vi "Main.vi"() -> ()   [LabVIEW 2015]
uses:
  <vilib>/myRIO/Instrument Drivers/Onboard IO/DIO/typedefs/DIO Reference.ctl
  <vilib>/myRIO/Common/Instrument Driver Framework/Utilities/typedefs/myRIO Generic Hardware Reference.ctl
  <vilib>/myRIO/Common/Instrument Driver Framework/Utilities/typedefs/Hardware Version Enum.ctl
  <vilib>/myRIO/Common/Instrument Driver Framework/Utilities/typedefs/myRIO v1.0 Reference.ctl
  <vilib>/myRIO/Common/Instrument Driver Framework/Utilities/typedefs/Generic FPGA Reference.ctl
  <vilib>/myRIO/Common/Instrument Driver Framework/myRIO v1.0/DIO/typedefs/DIO Channels List.ctl
  <vilib>/myRIO/Common/Instrument Driver Framework/myRIO v1.0/DIO/typedefs/DIO Channels Enum.ctl
  <vilib>/userdefined/High Color/nirio_resource_hc.ctl
  <vilib>/myRIO/Common/Instrument Driver Framework/Utilities/vis/Is FPGA Ref Available.vi
  <vilib>/myRIO/Common/Instrument Driver Framework/myRIO v1.0/DIO/vis/myRIO v1.1 Open DIO.vi
  <vilib>/myRIO/Instrument Drivers/Onboard IO/DIO/vis/Write.vi
  <vilib>/myRIO/Common/Instrument Driver Framework/Utilities/vis/Validate Channels.vi
  <vilib>/myRIO/Common/Instrument Driver Framework/myRIO v1.0/DIO/vis/myRIO v1.0 Reserve DIO.vi
  <vilib>/myRIO/Common/Instrument Driver Framework/myRIO v1.0/Resource Manager/vis/myRIO v1.0 Reserve Channel List.vi
  <vilib>/myRIO/Common/Instrument Driver Framework/myRIO v1.0/DIO/vis/myRIO v1.0 Build MUX Configuration DIO.vi
  <vilib>/myRIO/Common/Instrument Driver Framework/myRIO v1.0/Resource Manager/vis/myRIO v1.0 Reserve Channel.vi
  <vilib>/myRIO/Common/Instrument Driver Framework/myRIO v1.0/Resource Manager/vis/myRIO v1.0 Unreserve Channel.vi
  <vilib>/myRIO/Common/Instrument Driver Framework/myRIO v1.0/Resource Manager/vis/myRIO v1.0 Create Configuration List.vi
  <vilib>/myRIO/Common/Instrument Driver Framework/myRIO v1.0/Resource Manager/vis/myRIO v1.0 Build Mutex Name.vi
  <vilib>/Utility/VariantDataType/GetNumericInfo.vi
  <vilib>/Utility/error.llb/Error Cluster From Error Code.vi
  <vilib>/myRIO/Common/Instrument Driver Framework/myRIO v1.0/myRIO v1.1 Open.vi
  <vilib>/myRIO/Common/Instrument Driver Framework/Utilities/vis/IO Manager.vi
  <vilib>/myRIO/Common/Instrument Driver Framework/Utilities/vis/Configuration Manager.vi
  <vilib>/myRIO/Common/Instrument Driver Framework/myRIO v1.0/Resource Manager/vis/myRIO v1.0 Configure IO.vi
  <vilib>/myRIO/Common/Instrument Driver Framework/myRIO v1.0/myRIO v1.0 Close.vi
  <vilib>/myRIO/Common/Instrument Driver Framework/myRIO v1.0/DIO/vis/myRIO v1.0 Write DIO.vi
  <vilib>/myRIO/Express VI/Onboard Devices/LED/LED Express VI.xnode
  <vilib>/myRIO/Instrument Drivers/Onboard IO/DIO/vis/myRIO DIO Open.xnode
  <vilib>/myRIO/Express VI/Onboard IO/DO/DO Express VI.xnode
  <vilib>/myRIO/Instrument Drivers/Onboard IO/DIO/DIO.lvlib
panel:
  out "Image Out":T1(plugin-control)
  out "LMot":dbl(slide) scale=-1.0..1.0
  out "RMot":dbl(slide) scale=-1.0..1.0
  out "Translation Response":dbl
  out "Spin Response":dbl
  out "Y Axis Error":i32=100
  out "X Axis Error":i32=100
  out "Object Aquired":bool
  in  "stop":bool
  # "Robot Laser Tracker Main"
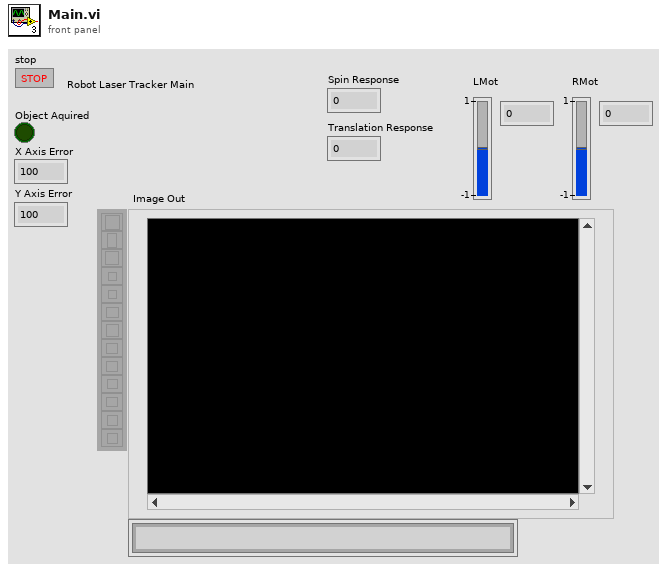
[diagram p1: front panel]
types:
  T1 = typedef "IMAQ Image.ctl" = refnum<image>
  T2 = typedef "DIO.lvlib/DIO Reference.ctl" = cluster{"myRIO Reference":T3, "DIO Channels List":T7}
  T3 = typedef "myRIO Generic Hardware Reference.ctl" = cluster{"myRIO Model":T4, "myRIO Hardware Reference":T5}
  T4 = typedef "Hardware Version Enum.ctl" = enum16{"Unknown", "myRIO-1900", "myRIO-1950", "roboRIO"}
  T5 = typedef "myRIO v1.0 Reference.ctl" = cluster{"Generic FPGA Reference":T6, "Allow multiple opens":bool}
  T6 = typedef "Generic FPGA Reference.ctl" = refnum<k20>
  T7 = typedef "DIO Channels List.ctl" = T8[]
  T8 = typedef "DIO Channels Enum.ctl" = enum16{"Not Connected", "C/DIO0", "C/DIO1", "C/DIO2", "C/DIO3", "C/DIO4", "C/DIO5", "C/DIO6", "C/DIO7", "A/DIO0", "A/DIO1", "A/DIO2", "A/DIO3", "A/DIO4", "A/DIO5", "A/DIO6", "A/DIO7", "A/DIO8", "A/DIO9", "A/DIO10", "A/DIO11", "A/DIO12", "A/DIO13", "A/DIO14", "A/DIO15", "B/DIO0", "B/DIO1", "B/DIO2", "B/DIO3", "B/DIO4", "B/DIO5", "B/DIO6", "B/DIO7", "B/DIO8", "B/DIO9", "B/DIO10", "B/DIO11", "B/DIO12", "B/DIO13", "B/DIO14", "B/DIO15", "LED0", "LED1", "LED2", "LED3", "Button0", "DIO/DIO0", "DIO/DIO1", "DIO/DIO2", "DIO/DIO3", "DIO/DIO4", "DIO/DIO5", "DIO/DIO6", "DIO/DIO7", "DIO/DIO8", "DIO/DIO9", "SPI/CS0", "SPI/CS1", "SPI/CS2", "SPI/CS3", "LED RADIO (Green)", "LED RADIO (Red)", "LED COMM (Green)", "LED COMM (Red)", "LED MODE (Green)", "LED MODE (Red)"}
  T9 = typedef "nirio_resource_hc.ctl" = tag
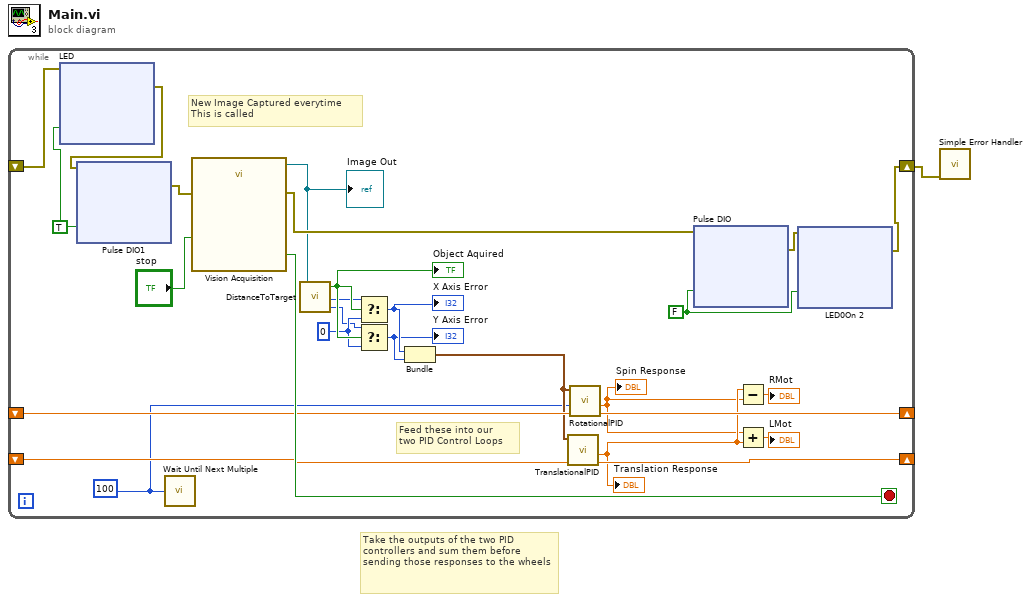
[diagram p0: block diagram]
diagram:
  # "Take the outputs of the two PID controllers and sum them before sending those responses to the wheels"
  n1 = while {
    shift-right: [w11] -> w1
    shift-left: _ -> [w14]
    shift-right: [w22] -> _
    shift-left: _ -> [w23]
    shift-right: [w21] -> _
    shift-left: _ -> [w20]
    stop <- w27 stop-if-true
    w5 = 0 ("f")
    w2 = u32 100 ("Tick Count(mSec)")
    w9 = FALSE ("A/DIO1 (Pin 13)")
    w12 = TRUE ("A/DIO1 (Pin 13)")
    # "New Image Captured everytime \nThis is called"
    # "Feed these into our \ntwo PID Control Loops"
    n2 = xnode "LED"("LED0"=w12, "error in (no error)"=w14) -> ("error out"=w13:errorcluster)
    n3 = xnode "Pulse DIO1"("A/DIO1 (Pin 13)"=w12, "error in (no error)"=w13) -> ("error out"=w28:errorcluster)
    n4 = call "Wait Until Next Multiple"("Count(mSec)"=w2) -> ()  [unwired: 1 out]
    n5 = call "Vision Acquisition"("Stop (F)"="stop", "error in"=w28) -> ("Image Out"=w24:T1, "Stopped"=w27:bool, "error out"=w25:errorcluster)  [unwired: 23 in]
    "Image Out" <- w24
    n6 = call "DistanceToTarget.vi"("Image Input"=w24) -> ("Y Axis Error"=w4:i32, "X Axis Error"=w6:i32, "Object Aquired"=w7:bool)  [unwired: 2 in]
    "Object Aquired" <- w7
    n7 = Select(t=w6, s=w7, f=w5) -> (s? t:f=w8:i32)
    "X Axis Error" <- w8
    n8 = Select(t=w4, s=w7, f=w5) -> (s? t:f=w3:i32)
    "Y Axis Error" <- w3
    n9 = Bundle("f"=w8, "f"=w3) -> (w19:cluster{"f":i32, "f":i32})  [unwired: 1 in]
    n10 = call "TranslationalPID.vi"("Old Error [pixels]"=w20, "DistanceToTarget [pixels]"=w19) -> ("New Error [pixels]"=w21:dbl, "Translation Response"=w16:dbl)  [unwired: 8 in]
    "Translation Response" <- w16
    n11 = call "RotationalPID.vi"("Old Error [radians]"=w23, "dTime [ms]"=w2, "DistanceToTarget [pixels]"=w19) -> ("New Error [radians]"=w22:dbl, "Spin Fraction Response"=w15:dbl)  [unwired: 7 in]
    "Spin Response" <- w15
    n12 = xnode "Pulse DIO"("A/DIO1 (Pin 13)"=w9, "error in (no error)"=w25) -> ("error out"=w10:errorcluster)
    n13 = Subtract(x=w16, y=w15) -> (x-y=→"RMot":dbl)
    n14 = Add(x=w15, y=w16) -> (x+y=→"LMot":dbl)
    n15 = xnode "LED0On 2"("LED0"=w9, "error in (no error)"=w10) -> ("error out"=w11:errorcluster)
  }
  n16 = call <vilib>:"Simple Error Handler.vi"("error in (no error)"=w1) -> ()  [unwired: 4 in, 5 out]
